vi "Error Queue Write.vi"(8 "error in (no error)":errorcluster) -> ()   [LabVIEW 2014]
panel:
  in  "timeout in ms (-1)":i32
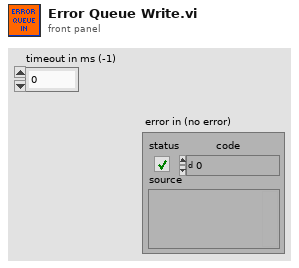
[diagram p1: front panel]
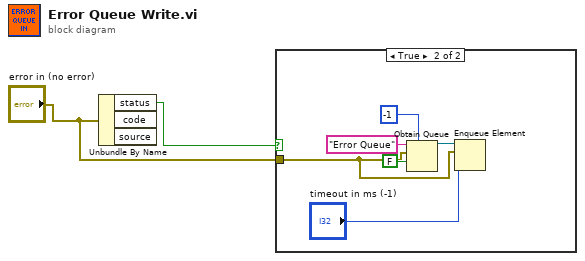
[diagram p0: block diagram]
diagram:
  n1 = Unbundle By Name("error in (no error)") -> ("status"=w2:bool)  [unwired: 2 out]
  n2 = case shown="True" w2 {
    tunnel: "error in (no error)" -> [_ w4]
    frame False {
    }
    frame True {
      n3 = Obtain Queue(max queue size (-1, unlimited)=-1, name (unnamed)="Error Queue", element data type=w4, create if not found? (T)=FALSE) -> (queue out=w5:refnum<queue>)  [unwired: 1 in, 2 out]
      n4 = Enqueue Element(queue=w5, element=w4, timeout in ms (-1)="timeout in ms (-1)") -> ()  [unwired: 1 in, 3 out]
    }
  }
